vi "gfitsio-create-file.vi"(8 "error in (no error)":errorcluster, 9 "overwrite? (F:no)":bool, 11 "path":path) -> (0 "error out":errorcluster, 3 "gfits refnum":T1)   [LabVIEW 2019, in "gfitsio.lvlib"]
doc: "Creates a new file and opens it for reading or writing. This function cannot overwrite an existing file unless overwrite is TRUE and the existing file is not read only. If you try to overwrite a file without the correct permission, this function does not create or open a file, and the function returns an error."
uses:
  gfitsio.lvlib
  gfitsio-refnum.ctl
  gfitsio.dll
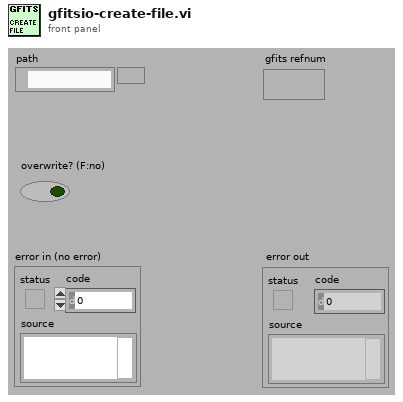
[diagram p1: front panel]
types:
  T1 = typedef "gfitsio.lvlib/gfitsio-refnum.ctl" = refnum<k1>
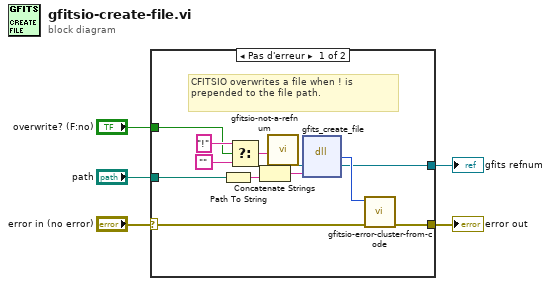
[diagram p0: block diagram]
diagram:
  n1 = case shown="Pas d'erreur" "error in (no error)" {
    selector: "error in (no error)" -> [w14 w18]
    tunnel: "path" -> [w17 _]
    tunnel: [w7 _] -> w4
    tunnel: [w15 w18] -> w3
    tunnel: "overwrite? (F:no)" -> [w8 _]
    frame No Error {
      # "CFITSIO overwrites a file when ! is prepended to the file path."
      n2 = Path To String(path=w17) -> (string=w13:string)
      n3 = Select(t="!", s=w8, f="") -> (s? t:f=w9:string)
      n4 = Concatenate Strings(w9, w13) -> (w12:string)
      n5 = call "gfitsio-not-a-refnum.vi"() -> ("invalid gfits refnum"=w6:T1)
      n6 = dll-call lib="C:/BonOMM_git/SubVIs/gfitsio/gfitsio.dll" fn="gfits_create_file"("invalid gfits refnum"=w6, "filename"=w12) -> (w16:i32, "invalid gfits refnum"=w7:T1)  [unwired: 4 in, 2 out]
      n7 = call "gfitsio-error-cluster-from-code.vi"("error in (no error)"=w14, "error code"=w16) -> ("error out"=w15:errorcluster)  [unwired: 9 in]
    }
    frame Error {
    }
  }
  "error out" <- w3
  "gfits refnum" <- w4
